vi "LabVIEW Type to JSON Tree.vi"() -> ()   [LabVIEW 2011]
uses:
  LabVIEW Type to JSON Tree Data.ctl
  i3-json.lvlib
panel:
  out "String":string
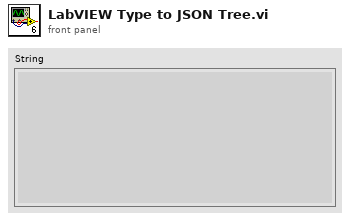
[diagram p1: front panel]
types:
  T1 = typedef "LabVIEW Type to JSON Tree Data.ctl" = cluster{"Zip Code":i32, "Name":string, "Is Awesome?":bool, "Products":cluster{"Product Name":string, "Serial Number":u32}[]}
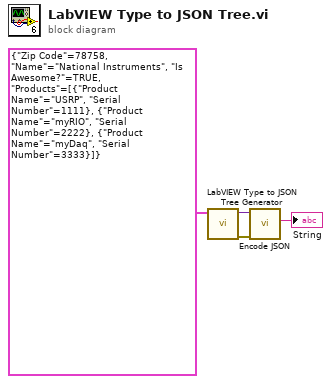
[diagram p0: block diagram]
diagram:
  n1 = call "LabVIEW Type to JSON Tree Generator.vi"("Cluster"=T1 {"Zip Code"=78758, "Name"="National Instruments", "Is Awesome?"=TRUE, "Products"=[{"Product Name"="USRP", "Serial Number"=1111}, {"Product Name"="myRIO", "Serial Number"=2222}, {"Product Name"="myDaq", "Serial Number"=3333}]}) -> ("error out"=w2:errorcluster, "JSON Tree Passthrough"=w3:variant)  [unwired: 9 in]
  n2 = call "Encode JSON.vi"("error in (no error)"=w2, "JSON Tree"=w3) -> ("String"=→"String":string)  [unwired: 4 in, 1 out]
